vi "does_obj_exist.vi"(10 "Plot Scene Object":refnum<vi>, 11 "Root":refnum<vi>) -> (2 "obj exists":bool)   [LabVIEW 2020, in "3DPC_SurfacePlot.xctl"]
uses:
  <vilib>/Native 3D Graph/xcontrol/3DPC_SurfacePlot.xctl
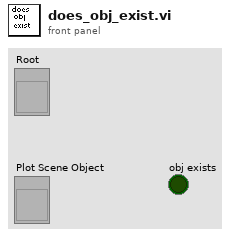
[diagram p1: front panel]
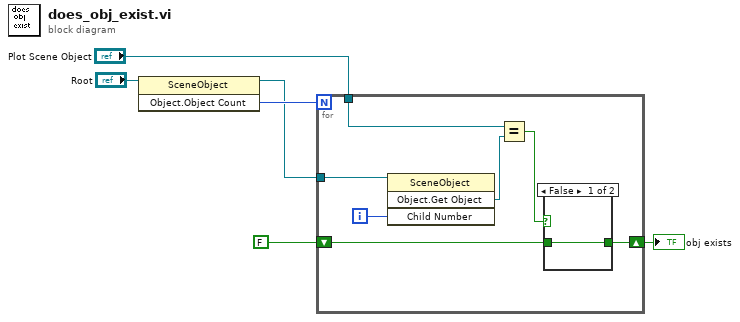
[diagram p0: block diagram]
diagram:
  n1 = invoke class="SceneObject" method="Object.Object Count"(reference="Root") -> (reference out=w5:refnum<vi>, "Child Count"=w6:i32)  [unwired: 2 in, 1 out]
  n2 = for {
    N: w6 -> [_]
    tunnel: w5 -> [w12]
    tunnel: "Plot Scene Object" -> [w11]
    shift-right: [w8] -> w1
    shift-left: FALSE -> [w7]
    i -> [w13]
    n3 = invoke class="SceneObject" method="Object.Get Object"(reference=w12, "Child Number"=w13) -> ("Get Child"=w10:refnum<vi>)  [unwired: 2 in, 3 out]
    n4 = Equal?(x=w11, y=w10) -> (x = y?=w9:bool)
    n5 = case shown="False" w9 {
      selector: w9 -> [_ w15]
      tunnel: [w14 w15] -> w8
      tunnel: w7 -> [w14 _]
      frame False {
      }
      frame True {
      }
    }
  }
  "obj exists" <- w1
